vi "Solve1.vi"(8 "Error In":errorcluster, 11 "object in":refnum<class "2021_11.lvclass">) -> (0 "Error Out":errorcluster, 2 "Result":u64, 3 "object out":refnum<class "2021_11.lvclass">)   [LabVIEW 2020, in "2021_11.lvclass"]
uses:
  2021_11.lvclass
  2021_11.lvclass/2021_11.ctl
  c093b6d8-f837-4f12-88b0-bb49c9534a44.vi
  c093b6d8-f837-4f12-88b0-bb49c9534a44.vi/be6f088c-3e4b-4523-ad48-2cdc85bad38a.vi
  c093b6d8-f837-4f12-88b0-bb49c9534a44.vi/f202eadf-433e-4cdb-b986-b2351ce8d73c.vi
  c093b6d8-f837-4f12-88b0-bb49c9534a44.vi/094751bc-bcf2-4346-afae-53942128b536.vi
  c093b6d8-f837-4f12-88b0-bb49c9534a44.vi/06ee343e-764f-4086-89d5-f578778d243c.vi
panel:
  out "Round":i32
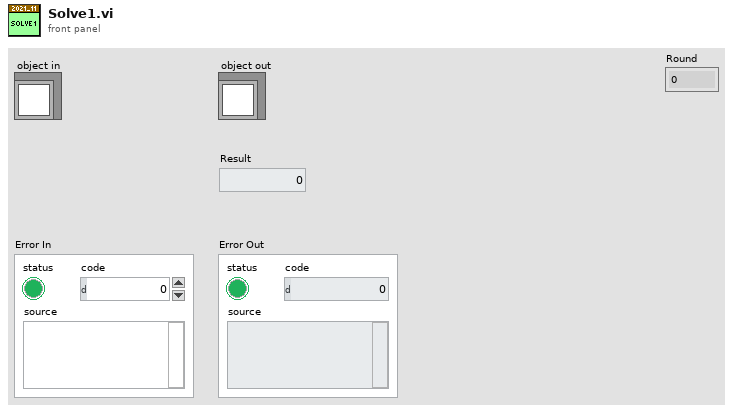
[diagram p1: front panel]
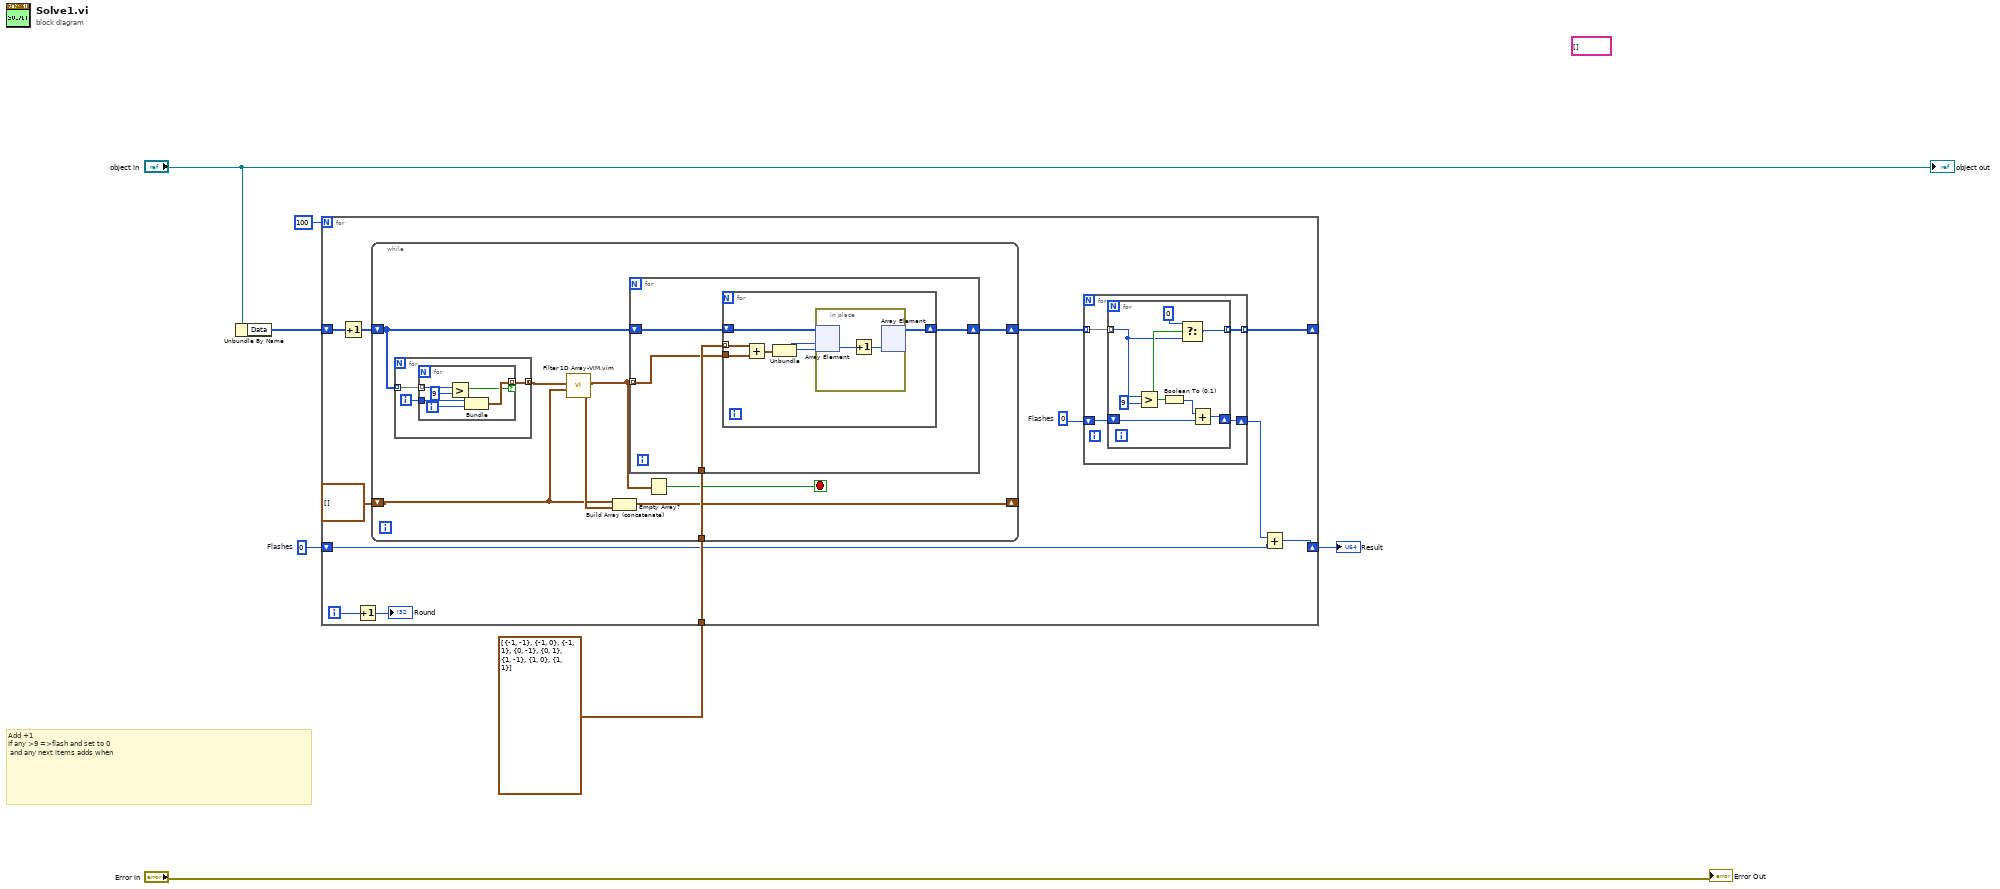
[diagram p0: block diagram]
diagram:
  w3 = 0  # Flashes
  (unwired) string[] [] ("LinesOfCode")
  # "Add +1\nIf any >9 =>flash and set to 0\n and any next items adds when"
  n1 = Unbundle By Name("object in") -> ("Data"=w5:i32[][])
  n2 = for {
    N: 100 -> [_]
    shift-right: [w9] -> _
    shift-left: w5 -> [w19]
    shift-right: [w10] -> w1
    shift-left: w3 -> [w12]
    tunnel: cluster{i32, i32}[] [{-1, -1}, {-1, 0}, {-1, 1}, {0, -1}, {0, 1}, {1, -1}, {1, 0}, {1, 1}] -> [w15]
    i -> [w18]
    w14 = 0  # Flashes
    n3 = Increment(x=w19) -> (x+1=w16:i32[][])
    n4 = Increment(x=w18) -> (x+1=→"Round":i32)
    n5 = while {
      tunnel: w15 -> [w26]
      shift-right: [w25] -> w13
      shift-left: w16 -> [w27]
      shift-right: [w22] -> _
      shift-left: cluster{i32, i32}[] [] -> [w20]
      stop <- w24 stop-if-true
      n6 = for {
        tunnel: w27 -> [w43] mode=indexing
        tunnel: [w41] -> w21 mode=concatenating
        i -> [w42]
        n7 = for {
          tunnel: w43 -> [w49] mode=indexing
          tunnel: w42 -> [w47]
          tunnel: [w45] -> w41 mode=indexing if=w44
          i -> [w46]
          n8 = Greater?(x=w49, y=9) -> (0:w44:bool)
          n9 = Bundle(w47, w46) -> (w45:cluster{i32, i32})  [unwired: 1 in]
        }
      }
      n10 = call "Filter 1D Array-VIM.vim"("Item(s) to Filter"=w20, "Array"=w21) -> ("Filtered Array"=w23:cluster{i32, i32}[])  [unwired: 5 in, 1 out]
      n11 = Build Array (concatenate)(w20, w23) -> (w22:cluster{i32, i32}[])
      n12 = for {
        tunnel: w23 -> [w29] mode=indexing
        shift-right: [w28] -> w25
        shift-left: w27 -> [w31]
        tunnel: w26 -> [w30]
        n13 = for {
          shift-right: [w32] -> w28
          shift-left: w31 -> [w36]
          tunnel: w30 -> [w38] mode=indexing
          tunnel: w29 -> [w37]
          n14 = Add(x=w38, y=w37) -> (x+y=w35:cluster{i32, i32})
          n15 = Unbundle(w35) -> (w34:i32, w33:i32)
          n16 = in-place {
            n17 = in-place-array #1(w36, w34, w33) -> (w40:i32)
            n18 = Increment(x=w40) -> (x+1=w39:i32)
            n19 = in-place-array #1(w39) -> (w32:i32[][])  [unwired: 2 out]
          }
        }
      }
      n20 = Empty Array?(array=w23) -> (empty?=w24:bool)
    }
    n21 = for {
      shift-right: [w51] -> w11
      shift-left: w14 -> [w53]
      tunnel: w13 -> [w52] mode=indexing
      tunnel: [w50] -> w9 mode=indexing
      n22 = for {
        shift-right: [w58] -> w51
        shift-left: w53 -> [w60]
        tunnel: w52 -> [w55] mode=indexing
        tunnel: [w54] -> w50 mode=indexing
        n23 = Greater?(x=w55, y=9) -> (0:w57:bool)
        n24 = Boolean To (0,1)(Boolean=w57) -> (0, 1=w59:i16)
        n25 = Select(t=0 ("y"), s=w57, f=w55) -> (s? t:f=w54:i32)
        n26 = Add(x=w59, y=w60) -> (x+y=w58:i32)
      }
    }
    n27 = Add(x=w11, y=w12) -> (x+y=w10:i32)
  }
  "Result" <- w1
  "Error Out" <- "Error In"
  "object out" <- "object in"
